vi "GLdrv_Close_USB.vi"(0 "hDevice":i32, 11 "error in (no error)":errorcluster) -> (15 "error out":errorcluster)   [LabVIEW 2017, in "GL860_Driver.lvlib"]
uses:
  GL860_Driver.lvlib
  gtcusbr.dll
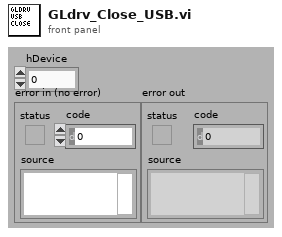
[diagram p1: front panel]
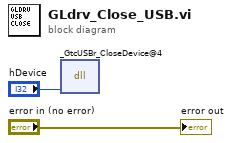
[diagram p0: block diagram]
diagram:
  n1 = dll-call lib="D:/src/LabVIEW/GL860/JP/LabView VI/Driver/gtcusbr.dll" fn="_GtcUSBr_CloseDevice@4"("HANDLE"="hDevice") -> ()  [unwired: 4 in, 3 out]
  "error out" <- "error in (no error)"
